vi "XNET Read (State Time Trigger).vi"(0 "session in":refnum<k21>, 9 "timeout (10)":dbl=10.0 format="%.2g", 11 "error in (no error)":errorcluster) -> (4 "session out":refnum<k21>, 6 "local time trigger":timestamp, 13 "network synced":bool, 14 "network time trigger":timestamp, 15 "error out":errorcluster)   [LabVIEW 2018]
doc: "Reads time at which the imported Time Trigger transitions low to high. The optional <B>timeout</B> can be used tio wait for the transition. The time is returned as a LabVIEW absolute timestamp. <B>local time communicating</B> uses the local timescale. <B>network time communicating</B> and <B>network synced</B> are applicable only for an Ethernet interface."
uses:
  nixlvapi.dll
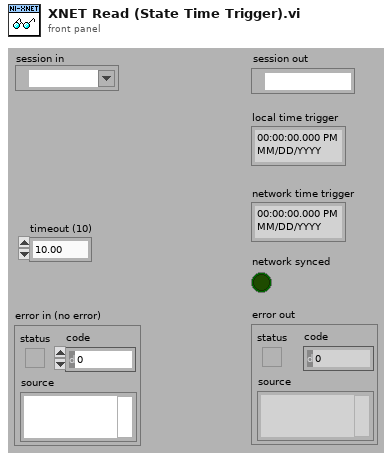
[diagram p1: front panel]
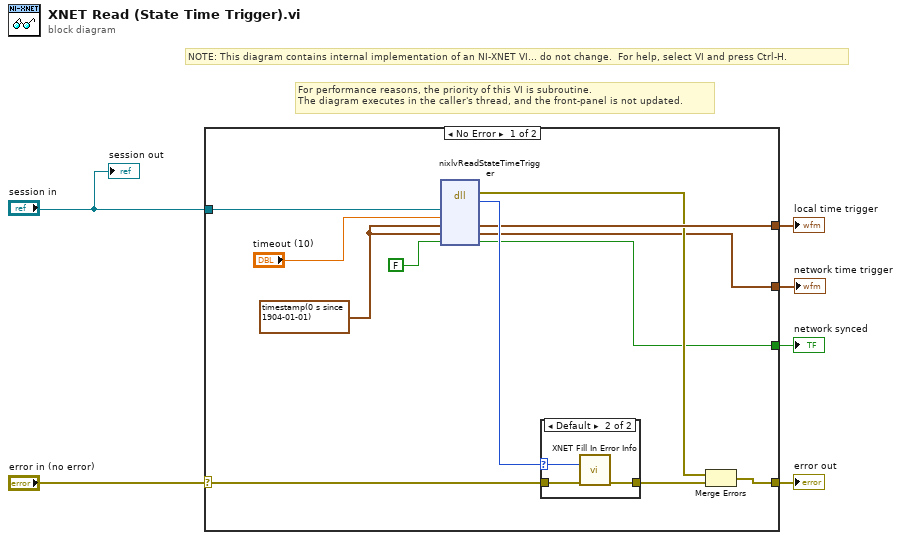
[diagram p0: block diagram]
diagram:
  # "For performance reasons, the priority of this VI is subroutine.\nThe diagram executes in the caller's thread, and the front-panel is not updated."
  # "NOTE: This diagram contains internal implementation of an NI-XNET VI... do not change.  For help, select VI and press Ctrl-H."
  n1 = case shown="No Error" "error in (no error)" {
    selector: "error in (no error)" -> [w17 w23]
    tunnel: "session in" -> [w18 _]
    tunnel: [w13 w23] -> w6
    tunnel: [w14 _] -> w3
    tunnel: [w8 _] -> w2
    tunnel: [w7 _] -> w1
    frame No Error {
      w11 = timestamp(0 s since 1904-01-01) ("time communication")
      n2 = dll-call lib="nixlvapi.*" fn="nixlvReadStateTimeTrigger"("sessionRef"=w18, "timeout"="timeout (10)", "localTime"=w11, "networkTime"=w11, "networkSynced"=FALSE ("network synced")) -> (error out=w12:errorcluster, "return type"=w15:i32, "localTime"=w14:timestamp, "networkTime"=w8:timestamp, "networkSynced"=w7:bool)  [unwired: 4 in, 2 out]
      n3 = case shown="Default" w15 {
        selector: w15 -> [_ w20]
        tunnel: w17 -> [w19 w21]
        tunnel: [w19 w22] -> w16
        frame 0 {
        }
        frame Default {
          n4 = call "XNET Fill In Error Info.vi"("status code"=w20, "error in"=w21) -> ("error out"=w22:errorcluster)  [unwired: 13 out]
        }
      }
      n5 = Merge Errors(w12, w16) -> (w13:errorcluster)
    }
    frame Error {
    }
  }
  "error out" <- w6
  "local time trigger" <- w3
  "network time trigger" <- w2
  "network synced" <- w1
  "session out" <- "session in"
